vi "sendValue.vi"(8 "error in (no error)":errorcluster, 10 "data":variant, 11 "stopShutter in":refnum<class "stopShutter.lvclass">) -> (0 "error out":errorcluster, 2 "function return":i32, 3 "stopShutter out":refnum<class "stopShutter.lvclass">)   [LabVIEW 2016, in "SALLV_AtDome_Messaging.lvlib" / "stopShutter.lvclass"]
uses:
  stopShutter.lvclass
  ts_sallv_AtDome/DataTypes/command_stopShutter.ctl
  ts_sallv_AtDome/SALLV_AtDome.lvlib
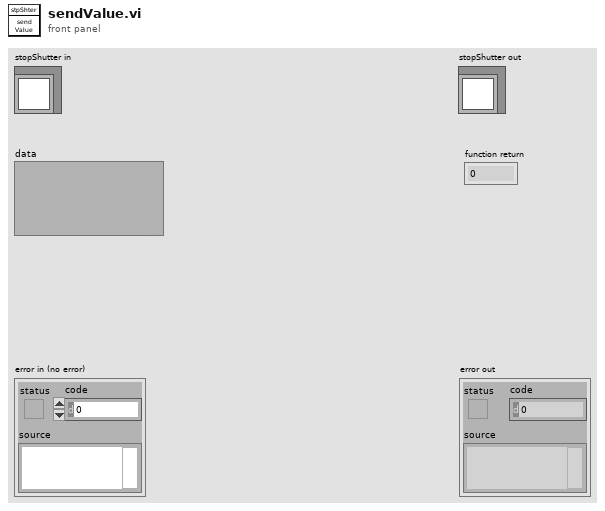
[diagram p1: front panel]
types:
  T1 = typedef "SALLV_AtDome.lvlib/command_stopShutter.ctl" = cluster{"value":bool}
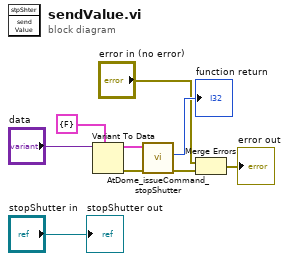
[diagram p0: block diagram]
diagram:
  n1 = Variant To Data(type=T1 {"value"=FALSE} ("command_stopShutter_Ctl"), Variant="data") -> (data=w6:T1, error out=w5:errorcluster)  [unwired: 1 in]
  n2 = call "AtDome_issueCommand_stopShutter.vi"("error in (no error)"=w5, "command_stopShutter_Ctl"=w6) -> ("error out"=w4:errorcluster, "function return"=→"function return":i32)  [unwired: 7 in, 1 out]
  n3 = Merge Errors("error in (no error)", w4) -> (→"error out":errorcluster)
  "stopShutter out" <- "stopShutter in"
